vi "Periodic Tasks.vi"() -> ()   [LabVIEW 2014]
doc: "This VI runs in parallel to other tasks. It can contain as many user-defined periodic loops as you need. These can carry out PID or other sorts of timed response."
uses:
  <vilib>/Rock Robotics/WPI/DriverStation/WPI_DriverStationRobotMode2.ctl
  NavX Code/navX-MXP Library/COMMON/TypeDefs/Value TypeDefs/navX Device Registers.ctl
  Global Variables.vi
  Robot Global Data.vi
  <vilib>/Utility/file.llb/Read From Spreadsheet File (DBL).vi
  <vilib>/Utility/file.llb/Write To Spreadsheet File (DBL).vi
  <vilib>/Rock Robotics/WPI/Joystick/WPI_JoystickGetSetRefNum.vi
  <vilib>/addons/control/pid/pid.llb/PID (DBL).vi
  <vilib>/addons/control/pid/NI_PID_pid.lvlib
  <vilib>/Rock Robotics/WPI/DriverStation/WPI_DriverStationStatusErrorCache.ctl
  NavX Code/navX-MXP Library/navX-MXP IMU.lvlib
panel:
  in  "Stationary Gryo":dbl
  in  "PID gains":T1={"proportional gain (Kc)"=0.02, "integral time (Ti, min)"=0.0, "derivative time (Td, min)"=0.0} {"derivative time (Td, min)" format="%.3f"; "integral time (Ti, min)" format="%.3f"; "proportional gain (Kc)" format="%.3f"}
  out "Valid?":bool
  out "Offset":dbl
  in  "Left Rumble":sgl
  in  "Right Rumble":sgl
  out "navX Data":u8[](array[numeric])
  in  "PID gains":T1={"proportional gain (Kc)"=1.0, "integral time (Ti, min)"=0.01, "derivative time (Td, min)"=0.0} {"derivative time (Td, min)" format="%.3f"; "integral time (Ti, min)" format="%.3f"; "proportional gain (Kc)" format="%.3f"}
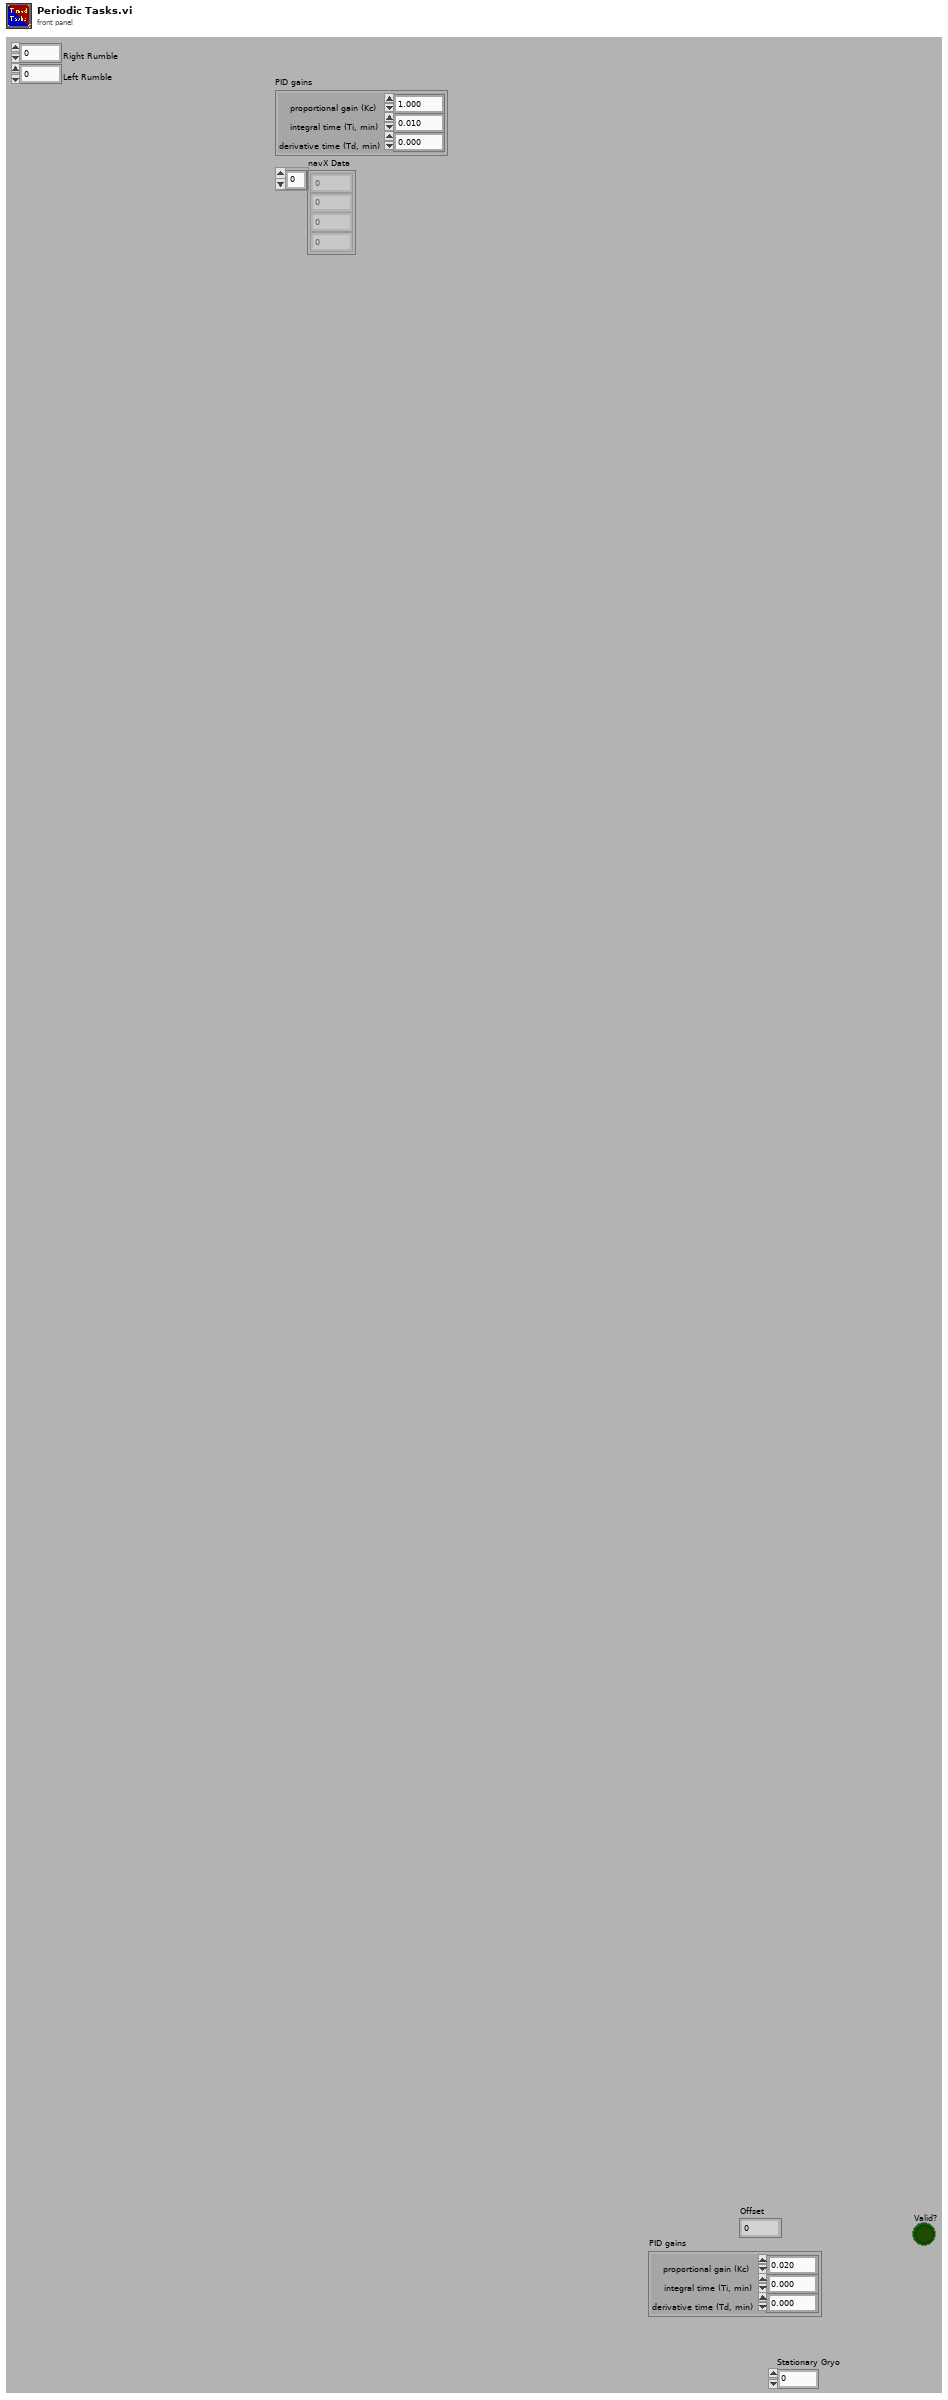
[diagram p1: front panel]
types:
  T1 = cluster{"proportional gain (Kc)":dbl, "integral time (Ti, min)":dbl, "derivative time (Td, min)":dbl}
  T2 = enum16{"Stop", "Three Tote", "Two Tote", "One Tote", "Step", "Top", "Home", "Joystick"}
  T3 = typedef "WPI_JoystickDevRef.ctl" = cluster{"Device":T4}
  T4 = typedef "WPI_JoystickDeviceEnum.ctl" = enum16{"USB 0", "USB 1", "USB 2", "USB 3", "USB 4", "USB 5"}
  T5 = typedef "WPI_DriverStationRobotMode2.ctl" = enum16{"Autonomous Disabled", "Autonomous Enabled", "Teleop Disabled", "Teleop Enabled", "Disconnected", "Finish", "Test Disabled", "Test Enabled", "Emergency Stopped"}
  T6 = typedef "navX-MXP IMU.lvlib/navX Device Registers.ctl" = u8
  T7 = typedef "navX-MXP IMU.lvlib/navX Device TypeDef.ctl" = cluster{"navX Interface Protocol":T8, "navX Interface Protocol TypeDefs":cluster{"SPIDevRef":T9, "I2CDevRef":T12}, "navX System Information":cluster{"Board Information":T14, "Status":T15, "Offsets":T19}, "navX Common Information":cluster{"Update Rate (4Hz-60Hz)":T20, "refnum name":string, "error":errorcluster}}
  T8 = typedef "navX-MXP IMU.lvlib/navX Interface Protocol.ctl" = enum16{"SPI", "I2C"}
  T9 = typedef "WPI_SPIDevRef.ctl" = cluster{"DevStatus":errorcluster, "Handle":i32, "Controller":T10, "SPI Bus":T11}
  T10 = typedef "FPGA_TypedefDigitalModule.ctl" = enum16{"Controller 1"}
  T11 = typedef "spi_bus.ctl" = enum16{"SPI On-Board, CS0", "SPI On-Board, CS1", "SPI On-Board, CS2", "SPI On-Board, CS3", "SPI MXP", "Invalid"}
  T12 = typedef "WPI_I2CDevRef.ctl" = cluster{"DevStatus":errorcluster, "Controller":T10, "Device Address":u8, "Handle":i32, "I2C Bus":T13}
  T13 = typedef "i2c_bus.ctl" = enum16{"I2C On-Board", "I2C MXP", "Invalid"}
  T14 = typedef "navX-MXP IMU.lvlib/navX Board Information.ctl" = cluster{"WhoAmI (50 | 0x32)":u8, "Board Revision":u8, "Firmware Major Version":u8, "Firmware Minor Version":u8}
  T15 = typedef "navX-MXP IMU.lvlib/navX Status Data.ctl" = cluster{"Update Rate Hz":u8, "Accelerometer Full-Scale Range":u8, "Gyro Full-Scale Range":u16, "NAVX_OP_STATUS":T16, "NAVX_CAL_STATUS":T17, "NAVX_SELFTEST_STATUS":u8, "NAVX_SENSOR_STATUS":T18}
  T16 = typedef "navX-MXP IMU.lvlib/navX NAVX_OP_STATUS.ctl" = u8
  T17 = typedef "navX-MXP IMU.lvlib/navX NAVX_CAL_STATUS.ctl" = u8
  T18 = typedef "navX-MXP IMU.lvlib/navX NAVX_SENSOR_STATUS.ctl" = cluster{"MOVING":bool, "YAW_STABLE":bool, "MAG_DISTURBANCE":bool, "ALTITUDE_VALID":bool, "SEALEVEL_PRESS_SET":bool, "FUSED_HEADING_VALID":bool}
  T19 = typedef "navX-MXP IMU.lvlib/navX Offsets Data.ctl" = cluster{"Yaw":dbl, "Quat W":dbl, "Quat X":dbl, "Quat Y":dbl, "Quat Z":dbl}
  T20 = typedef "navX-MXP IMU.lvlib/navX Update Rate.ctl" = u8
  T21 = typedef "WPI_DriverStationStatusErrorCache.ctl" = enum16{"Get", "Set"}
  T22 = typedef "WPI_MotorControlDeviceRef.ctl" = cluster{"DeviceStatus":errorcluster, "Type":T23, "PWM":cluster{"Controller":T10, "PWM Channel":T24, "DeadBand":T25}, "CAN":cluster{"Device Number":u8, "Control Mode":T26, "Semaphore":T27, "Max Vout":dbl, "TalonSRX Control Mode":T28}, "Invert":bool, "TransformRef":T29, "InvTransformRef":T29}
  T23 = typedef "WPI_MotorControlType.ctl" = enum16{"PWM", "CAN", "CANTalonSRX"}
  T24 = typedef "FPGA_DIOPWMChannel.ctl" = enum8{"PWM 0", "PWM 1", "PWM 2", "PWM 3", "PWM 4", "PWM 5", "PWM 6", "PWM 7", "PWM 8", "PWM 9", "PWM MXP 0", "PWM MXP 1", "PWM MXP 2", "PWM MXP 3", "PWM MXP 4", "PWM MXP 5", "PWM MXP 6", "PWM MXP 7", "PWM MXP 8", "PWM MXP 9", "Invalid"}
  T25 = typedef "WPI_PWMDeadband.ctl" = cluster{"Name":string, "maxPositivePwm":i32, "minPositivePwm":i32, "centerPwm":i32, "maxNegativePwm":i32, "minNegativePwm":i32, "angularRange":u16}
  T26 = typedef "WPI_CANJaguar_ControlMode.ctl" = enum8{"Percent VBus", "Current", "Speed", "Position", "Voltage"}
  T27 = typedef "Semaphore RefNum" = refnum<k1>
  T28 = typedef "WPI_CANTalonSRX_APIControlMode.ctl" = enum8{"Percent VBus", "Speed", "Position", "Slave", "Unchanged / Invalid"}
  T29 = typedef "WPI_PWMTransform_ConPane.ctl" = refnum<vi>
  T30 = typedef "WPI_CounterDevRef.ctl" = cluster{"DevStatus":errorcluster, "CntIndex":T31}
  T31 = typedef "FPGA_CounterCtrSystemIndex.ctl" = enum8{"Ctr 0", "Ctr 1", "Ctr 2", "Ctr 3", "Ctr 4", "Ctr 5", "Ctr 6", "Ctr 7", "Invalid"}
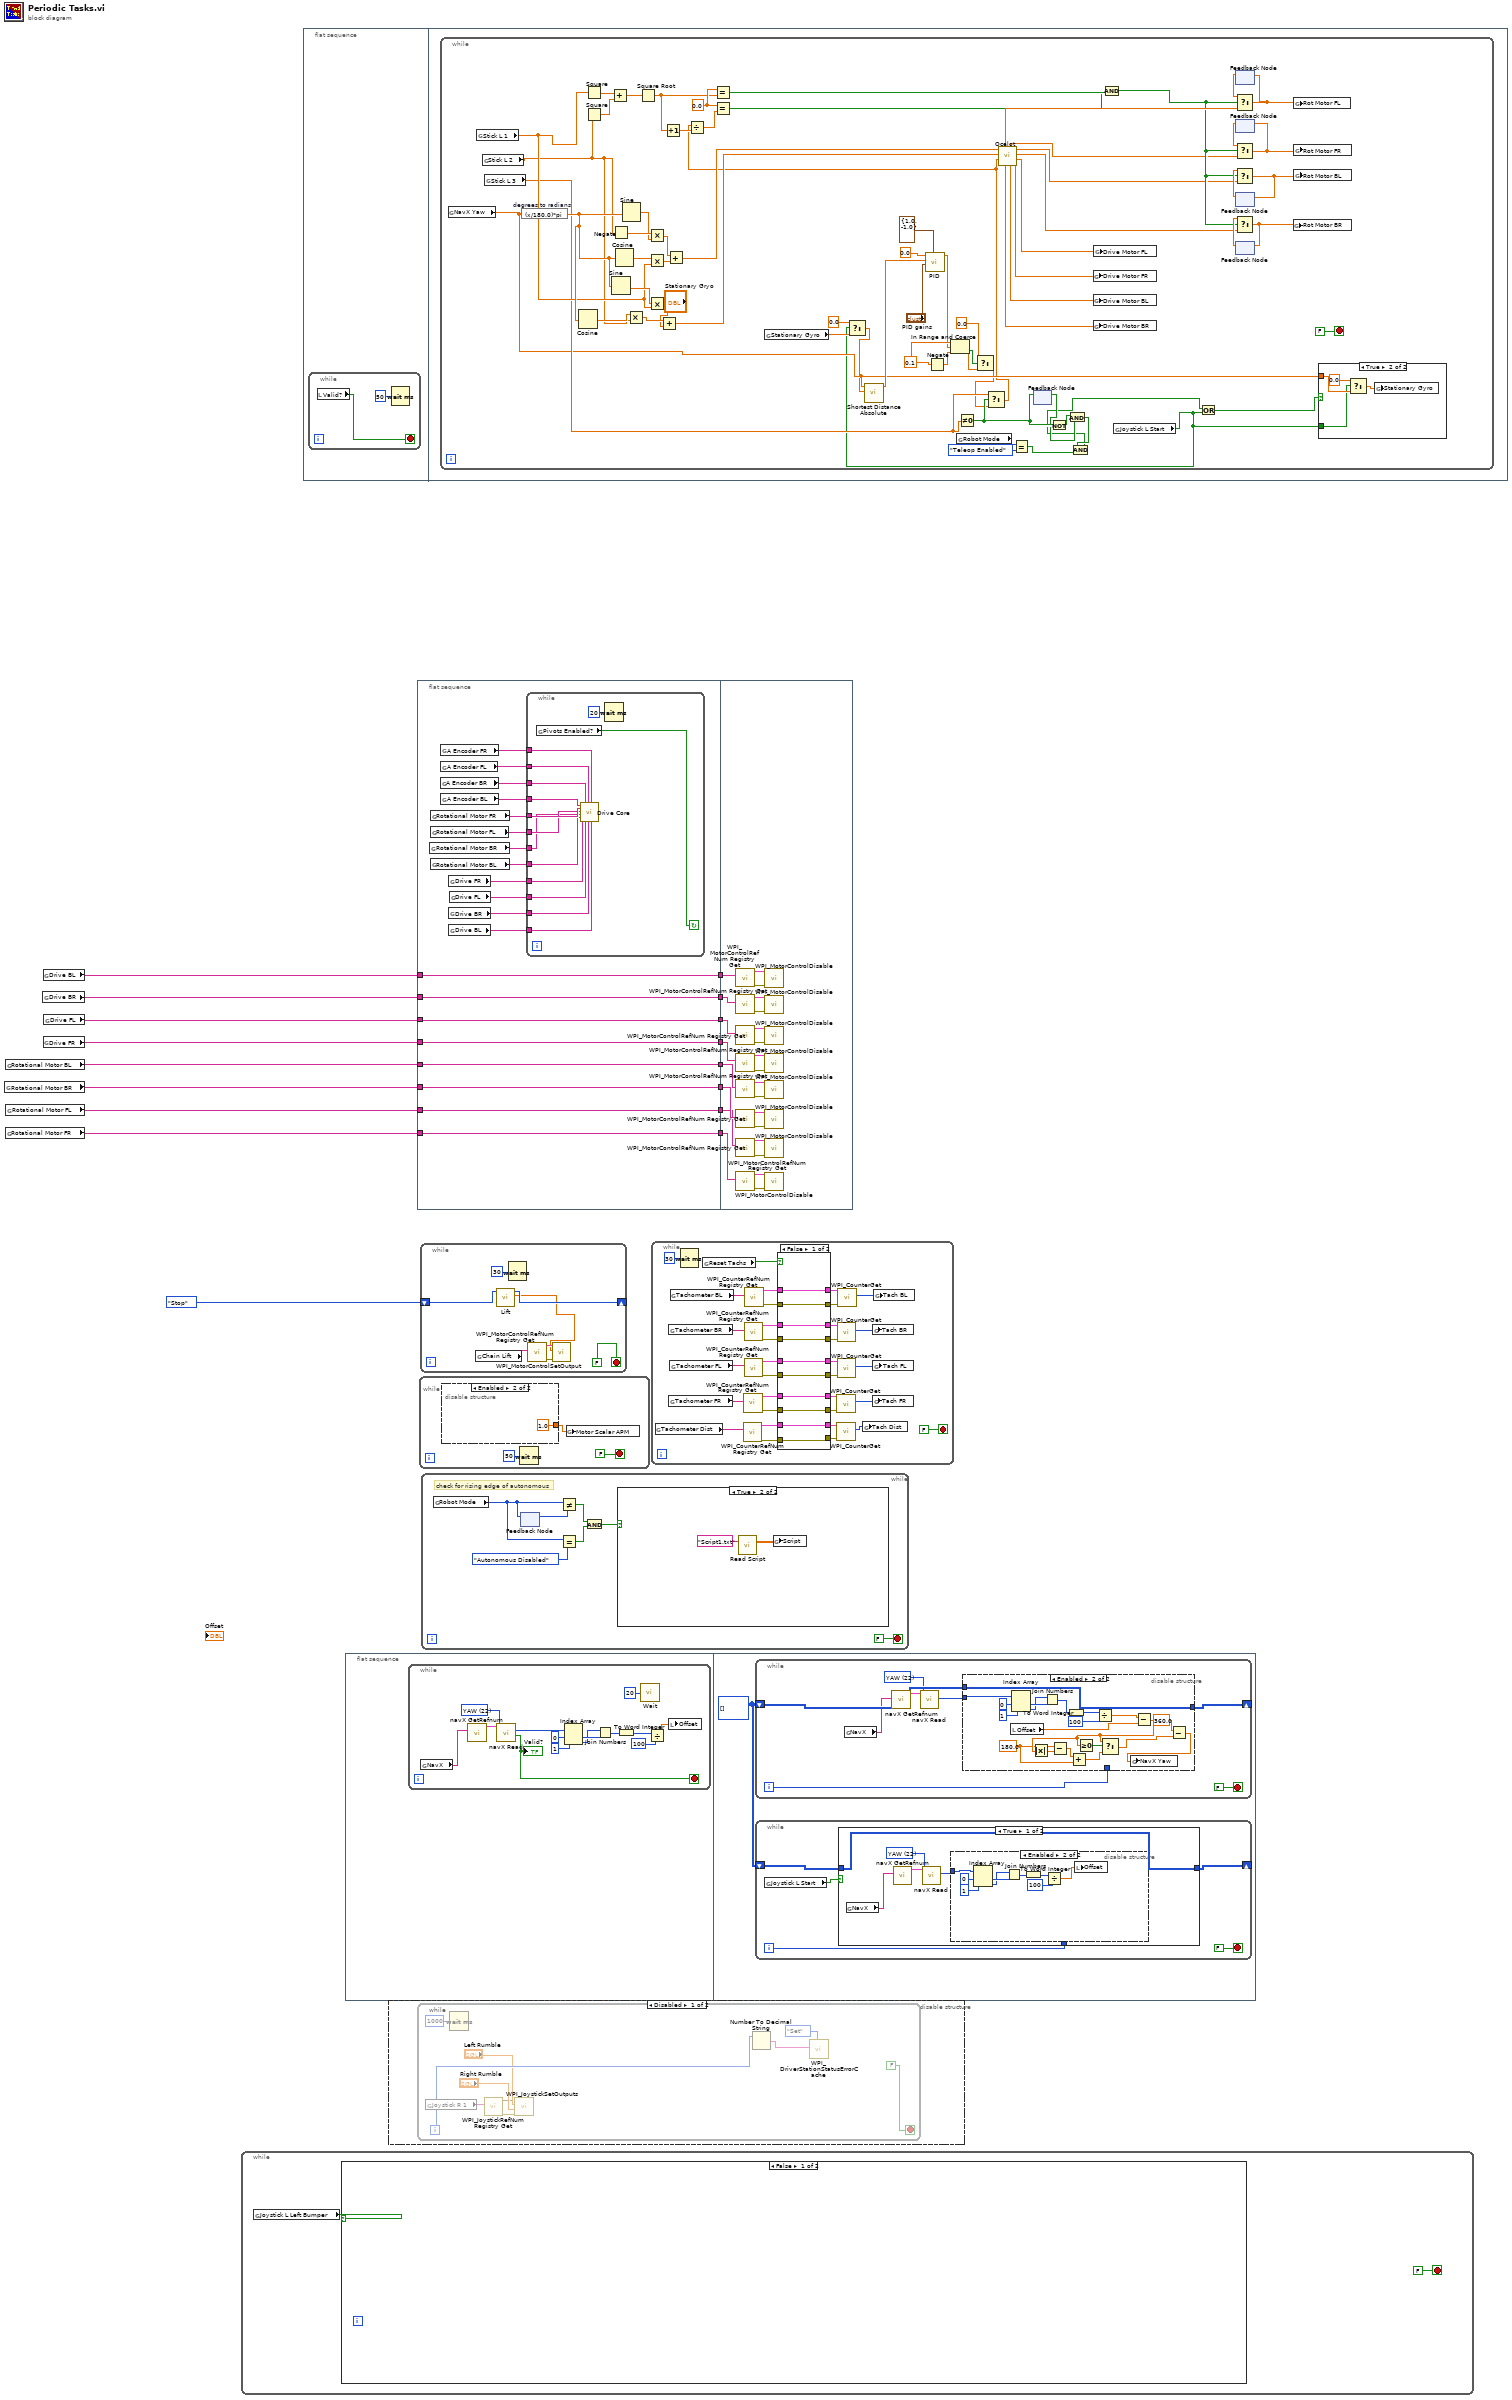
[diagram p0: block diagram]
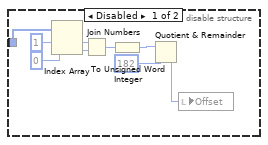
[diagram p3: hidden frame]
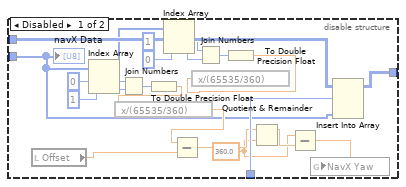
[diagram p5: hidden frame]
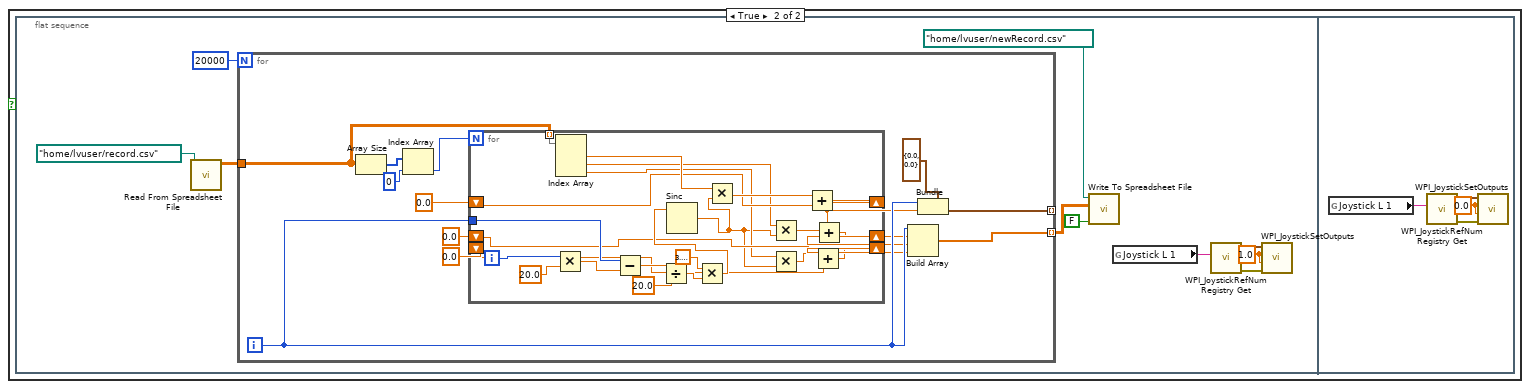
[diagram p6: hidden frame]
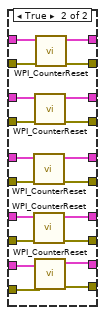
[diagram p9: hidden frame]
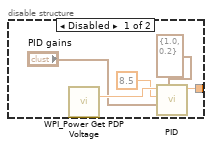
[diagram p10: hidden frame]
diagram:
  n1 = global read "Global Variables.vi" "Rotational Motor BR"() -> (w6:string)
  n2 = global read "Global Variables.vi" "Rotational Motor BL"() -> (w8:string)
  n3 = global read "Global Variables.vi" "Rotational Motor FR"() -> (w2:string)
  n4 = global read "Global Variables.vi" "Rotational Motor FL"() -> (w4:string)
  n5 = global read "Global Variables.vi" "Drive BR"() -> (w14:string)
  n6 = global read "Global Variables.vi" "Drive BL"() -> (w16:string)
  n7 = global read "Global Variables.vi" "Drive FR"() -> (w10:string)
  n8 = global read "Global Variables.vi" "Drive FL"() -> (w12:string)
  n9 = while {
    stop <- FALSE stop-if-true
    n10 = global read "Global Variables.vi" "Joystick L Left Bumper"() -> (w18:bool)
    n11 = case shown="False" w18 {
      frame False {
      }
      frame True {
        n12 = flat-sequence {
          frame #0 {
            w23 = sgl 1.0 ("Left Rumble")
            n13 = call-poly <vilib>:"Read From Spreadsheet File.vi"("file path (dialog if empty)"=path "/home/lvuser/record.csv") -> ("all rows"=w28:dbl[][])  [unwired: 6 in, 4 out]
            n14 = for {
              N: 20000 -> [_]
              tunnel: [w38] -> _ mode=indexing
              tunnel: w28 -> [w37]
              tunnel: [w34] -> w27 mode=indexing
              i -> [w36]
              n15 = Array Size(array=w37) -> (size(s)=w43:i32[])
              n16 = Index Array(array=w43, index=0) -> (element=w42:i32)
              n17 = for {
                N: w42 -> [_]
                shift-right: [w53] -> w35
                shift-left: 0.0 -> [w55]
                tunnel: w37 -> [w64] mode=indexing
                tunnel: w36 -> [w56]
                shift-right: [w51] -> w33
                shift-left: 0.0 -> [w48]
                shift-right: [w52] -> w32
                shift-left: 0.0 -> [w47]
                i -> [w62]
                n18 = Multiply(x=w62, y=20.0) -> (x*y=w59:dbl)
                n19 = Index Array(array=w64) -> (element #1=w65:dbl, element #2=w46:dbl, element #3=w45:dbl)  [unwired: 3 in]
                n20 = Subtract(x=w56, y=w59) -> (x-y=w61:dbl)
                n21 = Divide(x=w61, y=20.0) -> (x/y=w58:dbl)
                n22 = Multiply(x=3.141592653589793, y=w58) -> (x*y=w54:dbl)
                n23 = Sinc(1:w54) -> (0:w44:dbl)
                n24 = Multiply(x=w65, y=w44) -> (x*y=w66:dbl)
                n25 = Multiply(x=w46, y=w44) -> (x*y=w49:dbl)
                n26 = Multiply(x=w45, y=w44) -> (x*y=w50:dbl)
                n27 = Add(x=w66, y=w55) -> (x+y=w53:dbl)
                n28 = Add(x=w50, y=w47) -> (x+y=w52:dbl)
                n29 = Add(x=w49, y=w48) -> (x+y=w51:dbl)
              }
              n30 = Build Array(w36, w35, w33, w32) -> (w34:dbl[])
              n31 = Bundle(cluster=cluster{dbl, dbl} {0.0, 0.0}, w36, w35) -> (w38:cluster{dbl, dbl})
            }
            n32 = call-poly <vilib>:"Write To Spreadsheet File.vi"("append to file? (new file:F)"=FALSE, "2D data"=w27, "file path (dialog if empty)"=path "/home/lvuser/newRecord.csv") -> ()  [unwired: 5 in, 1 out]
            n33 = global read "Global Variables.vi" "Joystick L 1"() -> (w21:string)
            n34 = call <vilib>:"WPI_JoystickRefNum Registry Get.vi"("refnum name"=w21) -> ("error out"=w20:errorcluster, "JoystickDevRef"=w22:T3)  [unwired: 9 in]
            n35 = call <vilib>:"WPI_JoystickSetOutputs.vi"("error in (no error)"=w20, "Right Rumble"=w23, "Left Rumble"=w23, "JoystickDevRef"=w22) -> ()  [unwired: 6 in, 2 out]
          }
          frame #1 {
            w67 = sgl 0.0 ("Left Rumble")
            n36 = global read "Global Variables.vi" "Joystick L 1"() -> (w69:string)
            n37 = call <vilib>:"WPI_JoystickRefNum Registry Get.vi"("refnum name"=w69) -> ("error out"=w70:errorcluster, "JoystickDevRef"=w68:T3)  [unwired: 9 in]
            n38 = call <vilib>:"WPI_JoystickSetOutputs.vi"("error in (no error)"=w70, "Right Rumble"=w67, "Left Rumble"=w67, "JoystickDevRef"=w68) -> ()  [unwired: 6 in, 2 out]
          }
        }
      }
    }
  }
  n39 = flat-sequence {
    frame #0 {
      n40 = while {
        stop <- w72 stop-if-true
        n41 = local read "Valid?"() -> (w72:bool)
        n42 = Wait (ms)(milliseconds to wait=u32 50) -> ()  [unwired: 1 out]
      }
    }
    frame #1 {
      n43 = while {
        stop <- FALSE stop-if-true
        w83 = 0.1 ("Value to Deadband (default of 0.1)")
        w136 = 0.0 ("x")
        n44 = global read "Global Variables.vi" "NavX Yaw"() -> (w90:dbl)
        n45 = global read "Global Variables.vi" "Stick L 1"() -> (w97:dbl)
        n46 = global read "Global Variables.vi" "Stick L 2"() -> (w96:dbl)
        n47 = global read "Global Variables.vi" "Stick L 3"() -> (w95:dbl)
        n48 = expression code="(x/180.0)*pi" "degrees to radians"(w90) -> (w105:dbl)
        n49 = Cosine(x=w105) -> (cos(x)=w104:dbl)
        n50 = Square(x=w97) -> (x^2=w138:dbl)
        n51 = Square(x=w96) -> (x^2=w139:dbl)
        n52 = Add(x=w138, y=w139) -> (x+y=w137:dbl)
        n53 = Sine(x=w105) -> (sin(x)=w112:dbl)
        n54 = Negate(x=w96) -> (-x=w111:dbl)
        n55 = Cosine(x=w105) -> (cos(x)=w109:dbl)
        n56 = Sine(x=w105) -> (sin(x)=w106:dbl)
        n57 = Multiply(x=w104, y=w96) -> (x*y=w103:dbl)
        n58 = Square Root(x=w137) -> (sqrt(x)=w135:dbl)
        n59 = Multiply(x=w111, y=w106) -> (x*y=w110:dbl)
        n60 = Multiply(x=w109, y=w97) -> (x*y=w108:dbl)
        n61 = Multiply(x=w112, y=w97) -> (x*y=w102:dbl)
        n62 = Add(x=w103, y=w102) -> (x+y=w101:dbl)
        n63 = Increment(x=w135) -> (x+1=w134:dbl)
        n64 = Add(x=w110, y=w108) -> (x+y=w107:dbl)
        n65 = Equal?(x=w136, y=w135) -> (x = y?=w127:bool)
        n66 = global read "Global Variables.vi" "Stationary Gyro"() -> (w75:dbl)
        n67 = Negate(x=w83) -> (-x=w84:dbl)
        n68 = global read "Robot Global Data.vi" "Robot Mode"() -> (w88:T5)
        n69 = Not Equal To 0?(x=w95) -> (x != 0?=w92:bool)
        n70 = Equal?(x=w88, y=WPI_DriverStationRobotMode2."Teleop Enabled") -> (x = y?=w86:bool)
        n71 = feedback #1() -> (w91:bool)  [unwired: 1 in]
        n72 = feedback-in #1(w92) -> ()
        n73 = Not(x=w92) -> (.not. x?=w93:bool)
        n74 = And(x=w93, y=w91) -> (x .and. y?=w85:bool)
        n75 = And(x=w85, y=w86) -> (x .and. y?=w78:bool)
        n76 = global read "Global Variables.vi" "Joystick L Start"() -> (w73:bool)
        n77 = Select(t=0.0, s=w73, f=w75) -> (s? t:f=w76:dbl)
        n78 = call "Shortest Distance Absolute.vi"("Target"=w76, "Current"=w90) -> ("Angle to Rotate"=w94:dbl)  [unwired: 9 in]
        n79 = call-poly <vilib>:"PID.vi"("output range"=cluster{"output high":dbl, "output low":dbl} {"output high"=1.0, "output low"=-1.0}, "PID gains"="PID gains", "process variable"=w94, "setpoint"=0.0) -> ("output"=w80:dbl)  [unwired: 6 in, 1 out]
        n80 = In Range and Coerce(upper limit=w83, x=w80, lower limit=w84) -> (In Range?=w82:bool)  [unwired: 1 out]
        n81 = Select(t=0.0, s=w82, f=w80) -> (s? t:f=w79:dbl)
        n82 = Select(t=w95, s=w92, f=w79) -> (s? t:f=w89:dbl)
        n83 = Divide(x=w89, y=w134) -> (x/y=w133:dbl)
        n84 = Equal?(x=w136, y=w133) -> (x = y?=w126:bool)
        n85 = call "Ocelot.vi"("RCW (X2)"=w89, "FWD (Y)"=w101, "STR (X)"=w107) -> ("FRD"=w116:dbl, "FLD"=w117:dbl, "BRS"=w118:dbl, "BLS"=w119:dbl, "BLD"=w115:dbl, "FRS"=w120:dbl, "BRD"=w114:dbl, "FLS"=w128:dbl)  [unwired: 1 in]
        n86 = global write "Global Variables.vi" "Drive Motor FR"(w116) -> ()
        n87 = global write "Global Variables.vi" "Drive Motor BL"(w115) -> ()
        n88 = global write "Global Variables.vi" "Drive Motor BR"(w114) -> ()
        n89 = global write "Global Variables.vi" "Drive Motor FL"(w117) -> ()
        n90 = And(x=w127, y=w126) -> (x .and. y?=w125:bool)
        n91 = Or(x=w78, y=w73) -> (x .or. y?=w77:bool)
        n92 = feedback #2() -> (w132:dbl)  [unwired: 1 in]
        n93 = Select(t=w132, s=w125, f=w128) -> (s? t:f=w124:dbl)
        n94 = feedback-in #2(w124) -> ()
        n95 = feedback #3() -> (w131:dbl)  [unwired: 1 in]
        n96 = Select(t=w131, s=w125, f=w120) -> (s? t:f=w123:dbl)
        n97 = feedback-in #3(w123) -> ()
        n98 = feedback #4() -> (w130:dbl)  [unwired: 1 in]
        n99 = Select(t=w130, s=w125, f=w119) -> (s? t:f=w122:dbl)
        n100 = feedback-in #4(w122) -> ()
        n101 = feedback #5() -> (w129:dbl)  [unwired: 1 in]
        n102 = Select(t=w129, s=w125, f=w118) -> (s? t:f=w121:dbl)
        n103 = feedback-in #5(w121) -> ()
        n104 = global write "Global Variables.vi" "Rot Motor BR"(w121) -> ()
        n105 = global write "Global Variables.vi" "Rot Motor FL"(w124) -> ()
        n106 = global write "Global Variables.vi" "Rot Motor FR"(w123) -> ()
        n107 = global write "Global Variables.vi" "Rot Motor BL"(w122) -> ()
        n108 = case shown="True" w77 {
          tunnel: w90 -> [_ w142]
          tunnel: w73 -> [_ w140]
          frame False {
          }
          frame True {
            n109 = Select(t=0.0, s=w140, f=w142) -> (s? t:f=w143:dbl)
            n110 = global write "Global Variables.vi" "Stationary Gyro"(w143) -> ()
          }
        }
      }
    }
  }
  n111 = flat-sequence {
    frame #0 {
      n112 = while {
        stop <- w145 stop-if-true
        w157 = T6 22 items=["WHOAMI"=0, "HW_REV"=1, "FW_VER_MAJOR"=2, "FW_VER_MINOR"=3, "UPDATE_RATE_HZ"=4, "ACCEL_FSR_G"=5, "GYRO_FSR_DPS"=6, "OP_STATUS"=8, "CAL_STATUS"=9, "SELFTEST_STATUS"=10, "SENSOR_STATUS"=16, "TIMESTAMP"=18, "YAW"=22, "PITCH"=24, "ROLL"=26, "HEADING"=28, "FUSED_HEADING"=30, "ALTITUDE_I"=32, "ALTITUDE_D"=34, "LINERA_ACC_X"=36, "LINERA_ACC_Y"=38, "LINERA_ACC_Z"=40, "QUAT_W"=42, "QUAT_X"=44, "QUAT_Y"=46, "QUAT_Z"=48, "MPU_TEMP_C"=50, "GYRO_X"=52, "GYRO_Y"=54, "GYRO_Z"=56, "ACC_X"=58, "ACC_Y"=60, "ACC_Z"=62, "MAG_X"=64, "MAG_Y"=66, "MAG_Z"=68, "PRESSURE_I"=70, "PRESSURE_D"=72, "PRESSURE_TEMP"=74, "YAW_OFFSET"=76, "QUAT_OFFSET_W"=78, "QUAT_OFFSET_X"=80, "QUAT_OFFSET_Y"=82, "QUAT_OFFSET_Z"=84] ("Device Register (WHOAMI)")
        n113 = global read "Global Variables.vi" "NavX"() -> (w156:string)
        n114 = call "navX GetRefnum.vi"("refnum name"=w156) -> ("navX Device TypeDef"=w155:T7)  [unwired: 9 in, 1 out]
        n115 = call "navX Read.vi"("Device Register (WHOAMI)"=w157, "navX Device TypeDef"=w155) -> ("Valid?"=w145:bool, "navX Data"=w154:u8[])  [unwired: 7 in, 1 out]
        "Valid?" <- w145
        n116 = Index Array(array=w154, index #1=0 ("index"), index #2=1 ("index")) -> (element #1=w148:u8, element #2=w147:u8)
        n117 = Join Numbers(hi=w147, lo=w148) -> ((hi.lo)=w151:u16)
        n118 = To Word Integer(number=w151) -> (16bit integer=w150:i16)
        n119 = call "Wait"("Count(mSec)"=u32 20) -> ()  [unwired: 1 out]
        n120 = Divide(x=w150, y=i16 100) -> (x/y=w144:dbl)
        n121 = local write "Offset"(w144) -> ()
      }
    }
    frame #1 {
      w158 = u16[][] []
      n122 = while {
        shift-right: [w193] -> _
        shift-left: w158 -> [w192]
        i -> [w194]
        stop <- FALSE stop-if-true
        w189 = T6 22 items=["WHOAMI"=0, "HW_REV"=1, "FW_VER_MAJOR"=2, "FW_VER_MINOR"=3, "UPDATE_RATE_HZ"=4, "ACCEL_FSR_G"=5, "GYRO_FSR_DPS"=6, "OP_STATUS"=8, "CAL_STATUS"=9, "SELFTEST_STATUS"=10, "SENSOR_STATUS"=16, "TIMESTAMP"=18, "YAW"=22, "PITCH"=24, "ROLL"=26, "HEADING"=28, "FUSED_HEADING"=30, "ALTITUDE_I"=32, "ALTITUDE_D"=34, "LINERA_ACC_X"=36, "LINERA_ACC_Y"=38, "LINERA_ACC_Z"=40, "QUAT_W"=42, "QUAT_X"=44, "QUAT_Y"=46, "QUAT_Z"=48, "MPU_TEMP_C"=50, "GYRO_X"=52, "GYRO_Y"=54, "GYRO_Z"=56, "ACC_X"=58, "ACC_Y"=60, "ACC_Z"=62, "MAG_X"=64, "MAG_Y"=66, "MAG_Z"=68, "PRESSURE_I"=70, "PRESSURE_D"=72, "PRESSURE_TEMP"=74, "YAW_OFFSET"=76, "QUAT_OFFSET_W"=78, "QUAT_OFFSET_X"=80, "QUAT_OFFSET_Y"=82, "QUAT_OFFSET_Z"=84] ("Device Register (WHOAMI)")
        n123 = global read "Global Variables.vi" "NavX"() -> (w190:string)
        n124 = call "navX GetRefnum.vi"("refnum name"=w190) -> ("navX Device TypeDef"=w191:T7)  [unwired: 9 in, 1 out]
        n125 = call "navX Read.vi"("Device Register (WHOAMI)"=w189, "navX Device TypeDef"=w191) -> ("navX Data"=w188:u8[])  [unwired: 7 in, 2 out]
        n126 = disable-structure shown="Enabled" {
          disable-tunnel: w194 -> [w212 _]
          disable-tunnel: [w211 w236] -> w193
          disable-tunnel: w192 -> [w210 w236]
          disable-tunnel: w188 -> [w200 w237]
          frame Disabled {
            w206 = 360.0 ("y")
            n127 = local read "Offset"() -> (w209:dbl)
            n128 = Index Array(array=w200, index #1=0 ("index"), index #2=1 ("index")) -> (element #1=w217:u8, element #2=w216:u8)
            n129 = Join Numbers(hi=w217, lo=w216) -> ((hi.lo)=w213:u16)
            n130 = To Double Precision Float(number=w213) -> (double precision float=w204:dbl)
            n131 = expression code="x/(65535/360)"(w204) -> (w203:dbl)
            n132 = Index Array(array=w200, index #1=1 ("index"), index #2=0 ("index")) -> (element #1=w198:u8, element #2=w197:u8)
            n133 = Subtract(x=w203, y=w209) -> (x-y=w208:dbl)
            n134 = Join Numbers(hi=w198, lo=w197) -> ((hi.lo)=w199:u16)
            n135 = To Double Precision Float(number=w199) -> (double precision float=w196:dbl)
            n136 = expression code="x/(65535/360)"(w196) -> ()  [unwired: 1 out]
            n137 = Quotient & Remainder(x=w208, y=w206) -> (x-y*floor(x/y)=w207:dbl)  [unwired: 1 out]
            n138 = Subtract(x=w206, y=w207) -> (x-y=w205:dbl)
            n139 = global write "Global Variables.vi" "NavX Yaw"(w205) -> ()
            n140 = Insert Into Array(array=w210, index (row)=w212, new element=w200) -> (w211:u16[][])  [unwired: 1 in]
            "navX Data" <- w200
          }
          frame Enabled {
            w221 = 180.0 ("x")
            n141 = local read "Offset"() -> (w229:dbl)
            n142 = Index Array(array=w237, index #1=0 ("index"), index #2=1 ("index")) -> (element #1=w233:u8, element #2=w232:u8)
            n143 = Join Numbers(hi=w232, lo=w233) -> ((hi.lo)=w231:u16)
            n144 = To Word Integer(number=w231) -> (16bit integer=w228:i16)
            n145 = Divide(x=w228, y=i16 100) -> (x/y=w230:dbl)
            n146 = Subtract(x=w230, y=w229) -> (x-y=w225:dbl)
            n147 = Absolute Value(x=w225) -> (abs(x)=w224:dbl)
            n148 = Subtract(x=w221, y=w224) -> (x-y=w222:dbl)
            n149 = Add(x=w222, y=w221) -> (x+y=w223:dbl)
            n150 = Greater Or Equal To 0?(x=w225) -> (x >= 0?=w226:bool)
            n151 = Select(t=w225, s=w226, f=w223) -> (s? t:f=w219:dbl)
            n152 = Subtract(x=360.0, y=w219) -> (x-y=w218:dbl)
            n153 = global write "Global Variables.vi" "NavX Yaw"(w218) -> ()
          }
        }
      }
      n154 = while {
        shift-right: [w161] -> _
        shift-left: w158 -> [w160]
        i -> [w162]
        stop <- FALSE stop-if-true
        n155 = global read "Global Variables.vi" "Joystick L Start"() -> (w159:bool)
        n156 = case shown="True" w159 {
          tunnel: w162 -> [_ _]
          tunnel: [w164 w187] -> w161
          tunnel: w160 -> [w164 w187]
          frame True {
            w166 = T6 22 items=["WHOAMI"=0, "HW_REV"=1, "FW_VER_MAJOR"=2, "FW_VER_MINOR"=3, "UPDATE_RATE_HZ"=4, "ACCEL_FSR_G"=5, "GYRO_FSR_DPS"=6, "OP_STATUS"=8, "CAL_STATUS"=9, "SELFTEST_STATUS"=10, "SENSOR_STATUS"=16, "TIMESTAMP"=18, "YAW"=22, "PITCH"=24, "ROLL"=26, "HEADING"=28, "FUSED_HEADING"=30, "ALTITUDE_I"=32, "ALTITUDE_D"=34, "LINERA_ACC_X"=36, "LINERA_ACC_Y"=38, "LINERA_ACC_Z"=40, "QUAT_W"=42, "QUAT_X"=44, "QUAT_Y"=46, "QUAT_Z"=48, "MPU_TEMP_C"=50, "GYRO_X"=52, "GYRO_Y"=54, "GYRO_Z"=56, "ACC_X"=58, "ACC_Y"=60, "ACC_Z"=62, "MAG_X"=64, "MAG_Y"=66, "MAG_Z"=68, "PRESSURE_I"=70, "PRESSURE_D"=72, "PRESSURE_TEMP"=74, "YAW_OFFSET"=76, "QUAT_OFFSET_W"=78, "QUAT_OFFSET_X"=80, "QUAT_OFFSET_Y"=82, "QUAT_OFFSET_Z"=84] ("Device Register (WHOAMI)")
            n157 = global read "Global Variables.vi" "NavX"() -> (w167:string)
            n158 = call "navX GetRefnum.vi"("refnum name"=w167) -> ("navX Device TypeDef"=w168:T7)  [unwired: 9 in, 1 out]
            n159 = call "navX Read.vi"("Device Register (WHOAMI)"=w166, "navX Device TypeDef"=w168) -> ("navX Data"=w165:u8[])  [unwired: 7 in, 2 out]
            n160 = disable-structure shown="Enabled" {
              disable-tunnel: w165 -> [w172 w181]
              frame Disabled {
                n161 = Index Array(array=w172, index #1=1 ("index"), index #2=0 ("index")) -> (element #1=w171:u8, element #2=w170:u8)
                n162 = Join Numbers(hi=w171, lo=w170) -> ((hi.lo)=w175:u16)
                n163 = To Unsigned Word Integer(number=w175) -> (unsigned 16bit integer=w174:u16)
                n164 = Quotient & Remainder(x=w174, y=u16 182) -> (floor(x/y)=w169:u16)  [unwired: 1 out]
                n165 = local write "Offset"(w169) -> ()
              }
              frame Enabled {
                n166 = Index Array(array=w181, index #1=0 ("index"), index #2=1 ("index")) -> (element #1=w180:u8, element #2=w179:u8)
                n167 = Join Numbers(hi=w179, lo=w180) -> ((hi.lo)=w184:u16)
                n168 = To Word Integer(number=w184) -> (16bit integer=w183:i16)
                n169 = Divide(x=w183, y=i16 100) -> (x/y=w178:dbl)
                n170 = local write "Offset"(w178) -> ()
              }
            }
          }
          frame False {
          }
        }
      }
    }
  }
  n171 = disable-structure shown="Disabled" {
    frame Disabled {
      n172 = while {
        i -> [w244]
        stop <- FALSE stop-if-true
        n173 = global read "Global Variables.vi" "Joystick R 1"() -> (w239:string)
        n174 = Wait (ms)(milliseconds to wait=u32 1000) -> ()  [unwired: 1 out]
        n175 = call <vilib>:"WPI_JoystickRefNum Registry Get.vi"("refnum name"=w239) -> ("error out"=w238:errorcluster, "JoystickDevRef"=w240:T3)  [unwired: 9 in]
        n176 = call <vilib>:"WPI_JoystickSetOutputs.vi"("error in (no error)"=w238, "Right Rumble"="Right Rumble", "Left Rumble"="Left Rumble", "JoystickDevRef"=w240) -> ()  [unwired: 6 in, 2 out]
        n177 = Number To Decimal String(number=w244) -> (decimal integer string=w245:string)  [unwired: 1 in]
        n178 = call <vilib>:"WPI_DriverStationStatusErrorCache.vi"("StatusErrorCacheOp"=WPI_DriverStationStatusErrorCache."Set", "Error String"=w245) -> ()  [unwired: 1 in, 9 out]
      }
    }
    frame Enabled {
    }
  }
  n179 = flat-sequence {
    tunnel: [w255] -> w17
    tunnel: w16 -> [w255]
    tunnel: [w254] -> w15
    tunnel: w14 -> [w254]
    tunnel: [w253] -> w13
    tunnel: w12 -> [w253]
    tunnel: [w252] -> w11
    tunnel: w10 -> [w252]
    tunnel: [w251] -> w9
    tunnel: w8 -> [w251]
    tunnel: [w250] -> w7
    tunnel: w6 -> [w250]
    tunnel: [w249] -> w5
    tunnel: w4 -> [w249]
    tunnel: [w248] -> w3
    tunnel: w2 -> [w248]
    tunnel: w17 -> [w289]
    tunnel: w15 -> [w288]
    tunnel: w13 -> [w287]
    tunnel: w11 -> [w286]
    tunnel: w9 -> [w285]
    tunnel: w7 -> [w284]
    tunnel: w5 -> [w283]
    tunnel: w3 -> [w282]
    frame #0 {
      n180 = global read "Global Variables.vi" "Rotational Motor BR"() -> (w261:string)
      n181 = global read "Global Variables.vi" "Rotational Motor FR"() -> (w263:string)
      n182 = global read "Global Variables.vi" "Rotational Motor FL"() -> (w262:string)
      n183 = global read "Global Variables.vi" "Rotational Motor BL"() -> (w260:string)
      n184 = global read "Global Variables.vi" "A Encoder BR"() -> (w265:string)
      n185 = global read "Global Variables.vi" "A Encoder FR"() -> (w267:string)
      n186 = global read "Global Variables.vi" "A Encoder FL"() -> (w266:string)
      n187 = global read "Global Variables.vi" "A Encoder BL"() -> (w264:string)
      n188 = global read "Global Variables.vi" "Drive FR"() -> (w259:string)
      n189 = global read "Global Variables.vi" "Drive BR"() -> (w257:string)
      n190 = global read "Global Variables.vi" "Drive BL"() -> (w256:string)
      n191 = global read "Global Variables.vi" "Drive FL"() -> (w258:string)
      n192 = while {
        tunnel: w267 -> [w280]
        tunnel: w266 -> [w279]
        tunnel: w265 -> [w278]
        tunnel: w264 -> [w277]
        tunnel: w263 -> [w276]
        tunnel: w262 -> [w275]
        tunnel: w261 -> [w274]
        tunnel: w260 -> [w273]
        tunnel: w259 -> [w272]
        tunnel: w258 -> [w271]
        tunnel: w257 -> [w270]
        tunnel: w256 -> [w269]
        stop <- w281 continue-if-true
        n193 = global read "Global Variables.vi" "Pivots Enabled?"() -> (w281:bool)
        n194 = call "Drive Core.vi"("A Encoder BL"=w277, "Rotational Motor FR"=w276, "Rotational Motor FL"=w275, "Rotational Motor BR"=w274, "Rotational Motor BL"=w273, "Drive Motor FR"=w272, "A Encoder BR"=w278, "Drive Motor FL"=w271, "A Encoder FL"=w279, "Drive Motor BR"=w270, "A Encoder FR"=w280, "Drive Motor BL"=w269) -> ()  [unwired: 8 in]
        n195 = Wait (ms)(milliseconds to wait=u32 20) -> ()  [unwired: 1 out]
      }
    }
    frame #1 {
      n196 = call <vilib>:"WPI_MotorControlRefNum Registry Get.vi"("refnum name"=w289) -> ("error out"=w305:errorcluster, "MotorControlDevRef"=w304:T22)  [unwired: 9 in]
      n197 = call <vilib>:"WPI_MotorControlRefNum Registry Get.vi"("refnum name"=w288) -> ("error out"=w303:errorcluster, "MotorControlDevRef"=w302:T22)  [unwired: 9 in]
      n198 = call <vilib>:"WPI_MotorControlRefNum Registry Get.vi"("refnum name"=w287) -> ("error out"=w301:errorcluster, "MotorControlDevRef"=w300:T22)  [unwired: 9 in]
      n199 = call <vilib>:"WPI_MotorControlRefNum Registry Get.vi"("refnum name"=w286) -> ("error out"=w299:errorcluster, "MotorControlDevRef"=w298:T22)  [unwired: 9 in]
      n200 = call <vilib>:"WPI_MotorControlRefNum Registry Get.vi"("refnum name"=w285) -> ("error out"=w297:errorcluster, "MotorControlDevRef"=w296:T22)  [unwired: 9 in]
      n201 = call <vilib>:"WPI_MotorControlRefNum Registry Get.vi"("refnum name"=w284) -> ("error out"=w295:errorcluster, "MotorControlDevRef"=w294:T22)  [unwired: 9 in]
      n202 = call <vilib>:"WPI_MotorControlRefNum Registry Get.vi"("refnum name"=w283) -> ("error out"=w293:errorcluster, "MotorControlDevRef"=w292:T22)  [unwired: 9 in]
      n203 = call <vilib>:"WPI_MotorControlRefNum Registry Get.vi"("refnum name"=w282) -> ("error out"=w291:errorcluster, "MotorControlDevRef"=w290:T22)  [unwired: 9 in]
      n204 = call <vilib>:"WPI_MotorControlDisable.vi"("error in (no error)"=w305, "MotorControlDevRef"=w304) -> ()  [unwired: 8 in, 2 out]
      n205 = call <vilib>:"WPI_MotorControlDisable.vi"("error in (no error)"=w303, "MotorControlDevRef"=w302) -> ()  [unwired: 8 in, 2 out]
      n206 = call <vilib>:"WPI_MotorControlDisable.vi"("error in (no error)"=w301, "MotorControlDevRef"=w300) -> ()  [unwired: 8 in, 2 out]
      n207 = call <vilib>:"WPI_MotorControlDisable.vi"("error in (no error)"=w299, "MotorControlDevRef"=w298) -> ()  [unwired: 8 in, 2 out]
      n208 = call <vilib>:"WPI_MotorControlDisable.vi"("error in (no error)"=w297, "MotorControlDevRef"=w296) -> ()  [unwired: 8 in, 2 out]
      n209 = call <vilib>:"WPI_MotorControlDisable.vi"("error in (no error)"=w295, "MotorControlDevRef"=w294) -> ()  [unwired: 8 in, 2 out]
      n210 = call <vilib>:"WPI_MotorControlDisable.vi"("error in (no error)"=w293, "MotorControlDevRef"=w292) -> ()  [unwired: 8 in, 2 out]
      n211 = call <vilib>:"WPI_MotorControlDisable.vi"("error in (no error)"=w291, "MotorControlDevRef"=w290) -> ()  [unwired: 8 in, 2 out]
    }
  }
  n212 = while {
    stop <- FALSE stop-if-true
    n213 = disable-structure shown="Enabled" {
      disable-tunnel: [w309 1.0 ("Motor Scalar APM")] -> w306
      frame Disabled {
        n214 = call <vilib>:"WPI_Power Get PDP Voltage.vi"() -> ("voltage (V)"=w312:dbl)  [unwired: 14 in, 1 out]
        n215 = call-poly <vilib>:"PID.vi"("output range"=cluster{"output high":dbl, "output low":dbl} {"output high"=1.0, "output low"=0.2}, "PID gains"="PID gains", "process variable"=8.5 ("setpoint"), "setpoint"=w312) -> ("output"=w309:dbl)  [unwired: 6 in, 1 out]
      }
      frame Enabled {
      }
    }
    n216 = Wait (ms)(milliseconds to wait=u32 50) -> ()  [unwired: 1 out]
    n217 = global write "Global Variables.vi" "Motor Scalar APM"(w306) -> ()
  }
  n218 = while {
    shift-right: [w320] -> _
    shift-left: T2."Stop" ("State Out") -> [w321]
    stop <- FALSE stop-if-true
    n219 = global read "Global Variables.vi" "Chain Lift"() -> (w315:string)
    n220 = call "Lift.vi"("State"=w321) -> ("Lift Motor(Global...)"=w316:dbl, "State Out"=w320:T2)  [unwired: 9 in]
    n221 = Wait (ms)(milliseconds to wait=u32 30) -> ()  [unwired: 1 out]
    n222 = call <vilib>:"WPI_MotorControlRefNum Registry Get.vi"("refnum name"=w315) -> ("error out"=w319:errorcluster, "MotorControlDevRef"=w318:T22)  [unwired: 9 in]
    n223 = call <vilib>:"WPI_MotorControlSetOutput.vi"("error in (no error)"=w319, "Output"=w316, "MotorControlDevRef"=w318) -> ()  [unwired: 6 in, 3 out]
  }
  n224 = while {
    stop <- FALSE stop-if-true
    # "check for rising edge of autonomous"
    n225 = global read "Robot Global Data.vi" "Robot Mode"() -> (w327:T5)
    n226 = feedback #6() -> (w329:T5)  [unwired: 1 in]
    n227 = feedback-in #6(w327) -> ()
    n228 = Not Equal?(x=w327, y=w329) -> (x != y?=w325:bool)
    n229 = Equal?(x=w327, y=WPI_DriverStationRobotMode2."Autonomous Disabled" ("Robot Mode")) -> (x = y?=w326:bool)
    n230 = And(x=w325, y=w326) -> (x .and. y?=w323:bool)
    n231 = case shown="True" w323 {
      frame False {
      }
      frame True {
        n232 = call "Read Script.vi"("script name"="Script1.txt") -> ("output array"=w330:dbl[][])  [unwired: 1 in, 1 out]
        n233 = global write "Global Variables.vi" "Script"(w330) -> ()
      }
    }
  }
  n234 = while {
    stop <- FALSE stop-if-true
    n235 = global read "Global Variables.vi" "Tachometer Dist"() -> (w335:string)
    n236 = global read "Global Variables.vi" "Tachometer BR"() -> (w351:string)
    n237 = global read "Global Variables.vi" "Tachometer FR"() -> (w339:string)
    n238 = global read "Global Variables.vi" "Tachometer FL"() -> (w350:string)
    n239 = global read "Global Variables.vi" "Tachometer BL"() -> (w363:string)
    n240 = Wait (ms)(milliseconds to wait=u32 30) -> ()  [unwired: 1 out]
    n241 = global read "Global Variables.vi" "Reset Tachs"() -> (w362:bool)
    n242 = call <vilib>:"WPI_CounterRefNum Registry Get.vi"("refnum name"=w335) -> ("error out"=w333:errorcluster, "CounterDevRef"=w337:T30)  [unwired: 9 in]
    n243 = call <vilib>:"WPI_CounterRefNum Registry Get.vi"("refnum name"=w339) -> ("error out"=w341:errorcluster, "CounterDevRef"=w340:T30)  [unwired: 9 in]
    n244 = call <vilib>:"WPI_CounterRefNum Registry Get.vi"("refnum name"=w351) -> ("error out"=w353:errorcluster, "CounterDevRef"=w352:T30)  [unwired: 9 in]
    n245 = call <vilib>:"WPI_CounterRefNum Registry Get.vi"("refnum name"=w350) -> ("error out"=w348:errorcluster, "CounterDevRef"=w349:T30)  [unwired: 9 in]
    n246 = call <vilib>:"WPI_CounterRefNum Registry Get.vi"("refnum name"=w363) -> ("error out"=w360:errorcluster, "CounterDevRef"=w361:T30)  [unwired: 9 in]
    n247 = case shown="False" w362 {
      tunnel: w361 -> [w374 w394]
      tunnel: w360 -> [w373 w393]
      tunnel: [w374 w392] -> w359
      tunnel: [w373 w391] -> w358
      tunnel: w352 -> [w371 w381]
      tunnel: w353 -> [w372 w390]
      tunnel: [w371 w380] -> w354
      tunnel: [w372 w379] -> w355
      tunnel: w349 -> [w370 w382]
      tunnel: w348 -> [w369 w389]
      tunnel: [w370 w383] -> w347
      tunnel: [w369 w384] -> w346
      tunnel: w340 -> [w367 w387]
      tunnel: w341 -> [w368 w388]
      tunnel: [w367 w386] -> w342
      tunnel: [w368 w385] -> w343
      tunnel: w337 -> [w366 w378]
      tunnel: [w366 w377] -> w336
      tunnel: w333 -> [w365 w376]
      tunnel: [w365 w375] -> w332
      frame False {
      }
      frame True {
        n248 = call <vilib>:"WPI_CounterReset.vi"("error in (no error)"=w389, "CounterDevRef in"=w382) -> ("error out"=w384:errorcluster, "CounterDevRef out"=w383:T30)  [unwired: 8 in]
        n249 = call <vilib>:"WPI_CounterReset.vi"("error in (no error)"=w388, "CounterDevRef in"=w387) -> ("error out"=w385:errorcluster, "CounterDevRef out"=w386:T30)  [unwired: 8 in]
        n250 = call <vilib>:"WPI_CounterReset.vi"("error in (no error)"=w390, "CounterDevRef in"=w381) -> ("error out"=w379:errorcluster, "CounterDevRef out"=w380:T30)  [unwired: 8 in]
        n251 = call <vilib>:"WPI_CounterReset.vi"("error in (no error)"=w376, "CounterDevRef in"=w378) -> ("error out"=w375:errorcluster, "CounterDevRef out"=w377:T30)  [unwired: 8 in]
        n252 = call <vilib>:"WPI_CounterReset.vi"("error in (no error)"=w393, "CounterDevRef in"=w394) -> ("error out"=w391:errorcluster, "CounterDevRef out"=w392:T30)  [unwired: 8 in]
      }
    }
    n253 = call <vilib>:"WPI_CounterGet.vi"("error in (no error)"=w343, "CounterDevRef in"=w342) -> ("Value"=w344:i32)  [unwired: 4 in, 5 out]
    n254 = call <vilib>:"WPI_CounterGet.vi"("error in (no error)"=w332, "CounterDevRef in"=w336) -> ("Value"=w334:i32)  [unwired: 4 in, 5 out]
    n255 = call <vilib>:"WPI_CounterGet.vi"("error in (no error)"=w355, "CounterDevRef in"=w354) -> ("Value"=w356:i32)  [unwired: 4 in, 5 out]
    n256 = call <vilib>:"WPI_CounterGet.vi"("error in (no error)"=w346, "CounterDevRef in"=w347) -> ("Value"=w345:i32)  [unwired: 4 in, 5 out]
    n257 = call <vilib>:"WPI_CounterGet.vi"("error in (no error)"=w358, "CounterDevRef in"=w359) -> ("Value"=w357:i32)  [unwired: 4 in, 5 out]
    n258 = global write "Global Variables.vi" "Tach Dist"(w334) -> ()
    n259 = global write "Global Variables.vi" "Tach BR"(w356) -> ()
    n260 = global write "Global Variables.vi" "Tach FR"(w344) -> ()
    n261 = global write "Global Variables.vi" "Tach FL"(w345) -> ()
    n262 = global write "Global Variables.vi" "Tach BL"(w357) -> ()
  }
